vi "Waveform Circular Buffer.vi"(8 "error in":errorcluster, 9 "reset":bool, 10 "buffer duration (s)":dbl=10.0, 11 "waveform in":waveform(dbl)) -> (0 "error out":errorcluster, 3 "waveform out":waveform(dbl))   [LabVIEW 2019, in "DSP.lvclass"]
doc: "Circular buffer for the waveform datatype, designed for use with continuous data acquisition. The output is a single waveform with duration <b>buffer duration (s)</b>, in seconds. Input waveforms are appended to the end of the output waveform, and elements older than the buffer duration are discarded.\n\nAll input waveforms must have matching <i>dt</i> values. To eliminate drift in sample times, only the most recent trigger timestamp is considered; the trigger timestamp of the output waveform is computed from the most recently input trigger timestamp, the duration of the buffer, and <i>dt</i>. This may introduce jitter in sample times if the difference between the final timestamp of the previous input and the trigger timestamp of the next input are not exactly equal to <i>dt</i>. In this case, the timestamps of the most recent portion of the buffer will be correct, but earlier timestamps will be scaled. In buffered continuous acquisition, waveforms are consecutive and no jitter is introduced by this method.\n\nThe duration of the buffer may be larger than the requested duration if the duration is not an integer multiple of <i>dt</i>.\n\nOn first call, the input waveform fills end of the buffer; earlier values are set to zero, and the trigger timestamp is backdated. For performance reasons, <b>buffer duration (s)</b> is read only on first call."
uses:
  DSP.lvclass
  <vilib>/Waveform/WDTOps.llb/WDT Number of Waveform Samples DBL.vi
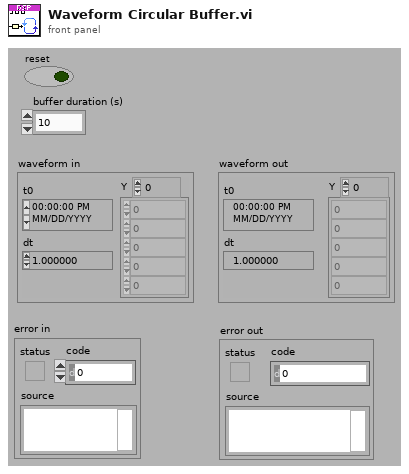
[diagram p1: front panel]
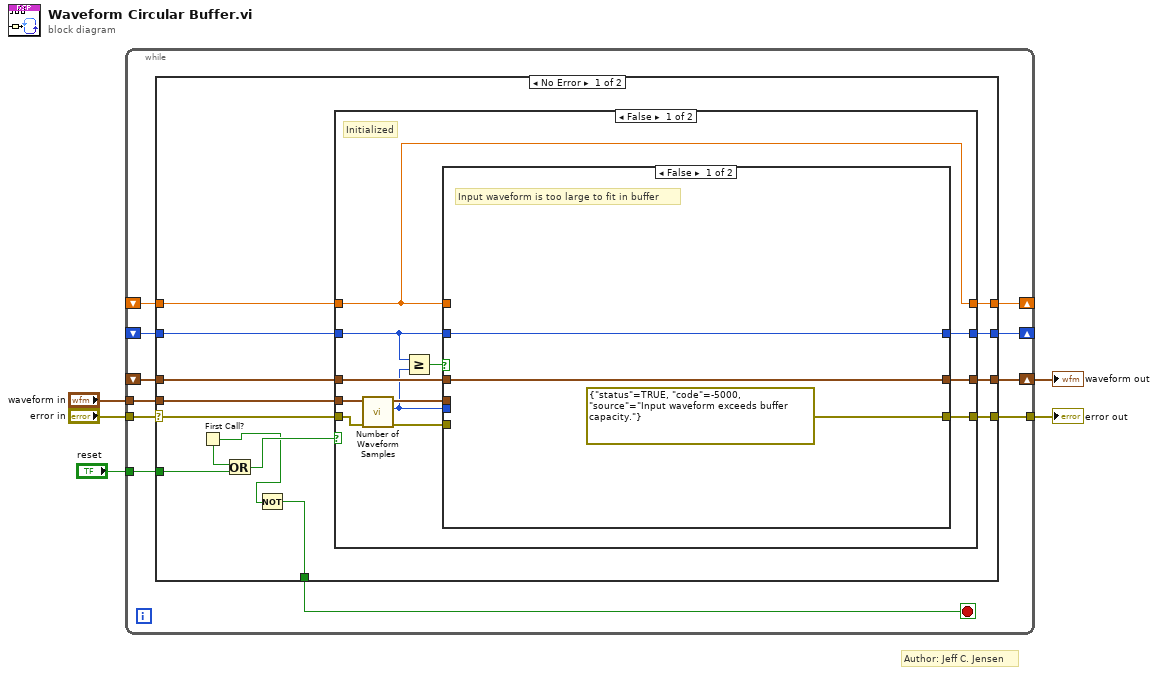
[diagram p0: block diagram]
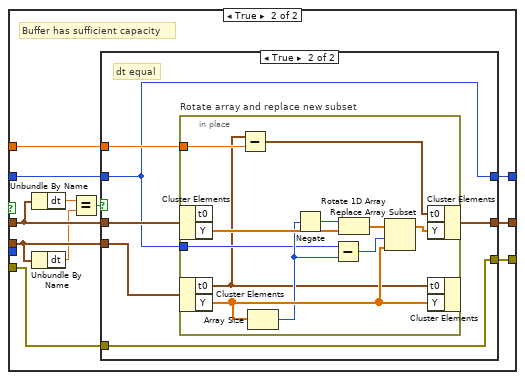
[diagram p2: hidden frame]
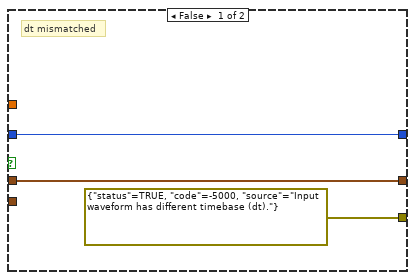
[diagram p3: hidden frame]
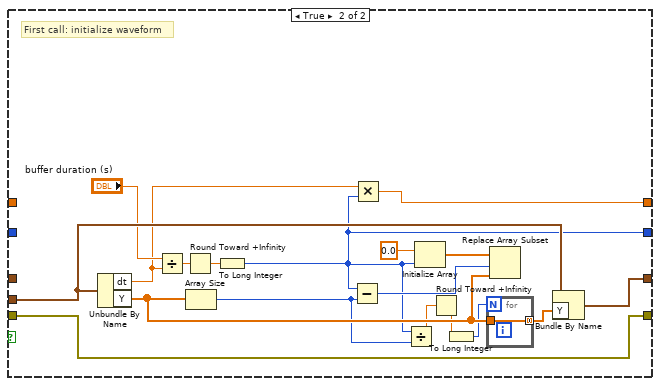
[diagram p4: hidden frame]
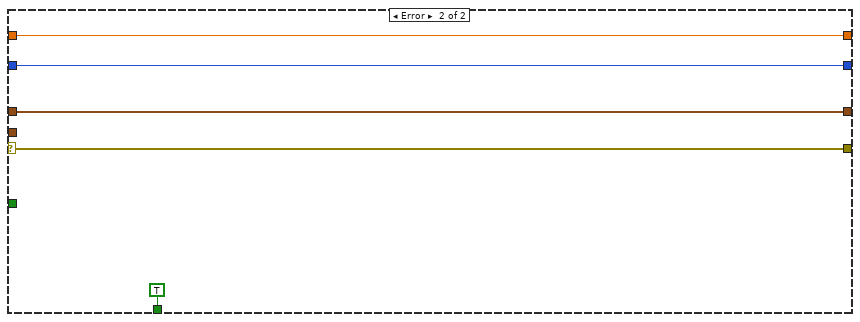
[diagram p5: hidden frame]
diagram:
  # "Author: Jeff C. Jensen"
  n1 = while {
    tunnel: "waveform in" -> [w16]
    tunnel: "error in" -> [w8]
    tunnel: [w14] -> w3
    shift-right: [w15] -> w4
    shift-left: _ -> [w13]
    shift-right: [w12] -> _
    shift-left: _ -> [w11]
    shift-right: [w10] -> _
    shift-left: _ -> [w9]
    tunnel: "reset" -> [w6]
    stop <- w7 stop-if-true
    n2 = case shown="No Error" w8 {
      selector: w8 -> [w21 w95]
      tunnel: w16 -> [w29 _]
      tunnel: [w28 w98] -> w15
      tunnel: [w20 TRUE ("First Call?: T/F")] -> w7
      tunnel: [w27 w95] -> w14
      tunnel: w13 -> [w26 w98]
      tunnel: [w25 w97] -> w12
      tunnel: w11 -> [w24 w97]
      tunnel: [w23 w96] -> w10
      tunnel: w9 -> [w22 w96]
      tunnel: w6 -> [w19 _]
      frame No Error {
        n3 = First Call?() -> (First Call?: T/F=w17:bool)
        n4 = Or(x=w17, y=w19) -> (x .or. y?=w18:bool)
        n5 = Not(x=w17) -> (.not. x?=w20:bool)
        n6 = case shown="False" w18 {
          tunnel: w29 -> [w38 w92]
          tunnel: [w41 w91] -> w28
          tunnel: w21 -> [w37 w90]
          tunnel: [w40 w90] -> w27
          tunnel: w26 -> [w39 _]
          tunnel: [w34 w79] -> w25
          tunnel: w24 -> [w30 _]
          tunnel: [w33 w83] -> w23
          tunnel: w22 -> [w33 _]
          frame False {
            # "Initialized"
            n7 = call-poly <vilib>:"Number of Waveform Samples.vi"("error in (no error)"=w37, "waveform in"=w38) -> ("error out"=w36:errorcluster, "number of samples"=w31:i32, "waveform out"=w35:waveform(dbl))  [unwired: 7 in]
            n8 = Greater Or Equal?(x=w30, y=w31) -> (x >= y?=w32:bool)
            n9 = case shown="False" w32 {
              tunnel: [w44 w55] -> w41
              tunnel: [errorcluster {"status"=TRUE, "code"=-5000, "source"="Input waveform exceeds buffer capacity."} ("error out") w47] -> w40
              tunnel: w39 -> [w44 w51]
              tunnel: w36 -> [_ w46]
              tunnel: w35 -> [_ w52]
              tunnel: w31 -> [_ _]
              tunnel: w30 -> [w43 w54]
              tunnel: [w43 w48] -> w34
              tunnel: w33 -> [_ w53]
              frame False {
                # "Input waveform is too large to fit in buffer"
              }
              frame True {
                # "Buffer has sufficient capacity"
                n10 = Unbundle By Name(w51) -> ("dt"=w50:dbl)
                n11 = Unbundle By Name(w52) -> ("dt"=w49:dbl)
                n12 = Equal?(x=w50, y=w49) -> (x = y?=w45:bool)
                n13 = case shown="True" w45 {
                  tunnel: [w57 w64] -> w55
                  tunnel: w51 -> [w57 w63]
                  tunnel: w52 -> [_ w62]
                  tunnel: w54 -> [w58 w60]
                  tunnel: w53 -> [_ w61]
                  tunnel: [w58 w60] -> w48
                  tunnel: [errorcluster {"status"=TRUE, "code"=-5000, "source"="Input waveform has different timebase (dt)."} ("error out") w59] -> w47
                  tunnel: w46 -> [_ w59]
                  frame False {
                    # "dt mismatched"
                  }
                  frame True {
                    # "dt equal"
                    n14 = in-place "Rotate array and replace new subset" {
                      in-place-border: w60 -> [w68]
                      in-place-border: w61 -> [w66]
                      n15 = in-place-cluster #1(w63) -> ("Y"=w72:dbl[])  [unwired: 1 out]
                      n16 = in-place-cluster #2(w62) -> ("t0"=w65:timestamp, "Y"=w70:dbl[])
                      n17 = Subtract(x=w65, y=w66) -> (x-y=w67:timestamp)
                      n18 = Array Size(array=w70) -> (size(s)=w69:i32)
                      n19 = Negate(x=w69) -> (-x=w73:i32)
                      n20 = Subtract(x=w68, y=w69) -> (x-y=w71:i32)
                      n21 = Rotate 1D Array(1:w72, 2:w73) -> (0:w75:dbl[])
                      n22 = Replace Array Subset(array=w75, new element=w70, index=w71) -> (w74:dbl[])
                      n23 = in-place-cluster #1("t0"=w67, "Y"=w74) -> (w64:waveform(dbl))
                      n24 = in-place-cluster #2("t0"=w65, "Y"=w70) -> ()  [unwired: 1 out]
                    }
                  }
                }
              }
            }
          }
          frame True {
            # "First call: initialize waveform"
            n25 = Unbundle By Name(w92) -> ("dt"=w84:dbl, "Y"=w81:dbl[])
            n26 = Divide(x="buffer duration (s)", y=w84) -> (x/y=w86:dbl)
            n27 = Round Toward +Infinity(x=w86) -> (ceil(x): smallest int >= x=w85:dbl)
            n28 = Array Size(array=w81) -> (size(s)=w80:i32)
            n29 = To Long Integer(number=w85) -> (32bit integer=w79:i32)
            n30 = Subtract(x=w79, y=w80) -> (x-y=w89:i32)
            n31 = Multiply(x=w84, y=w79) -> (x*y=w83:dbl)
            n32 = Divide(x=w79, y=w80) -> (x/y=w78:dbl)
            n33 = Initialize Array(0.0, w79) -> (w88:dbl[])
            n34 = Round Toward +Infinity(x=w78) -> (ceil(x): smallest int >= x=w77:dbl)
            n35 = To Long Integer(number=w77) -> (32bit integer=w76:i32)
            n36 = for {
              N: w76 -> [_]
              tunnel: [w94] -> w82 mode=concatenating
              tunnel: w81 -> [w94]
            }
            n37 = Replace Array Subset(array=w88, new element=w81, index=w89) -> ()  [unwired: 1 out]
            n38 = Bundle By Name(cluster=w92, "Y"=w82) -> (w91:waveform(dbl))
          }
        }
      }
      frame Error {
      }
    }
  }
  "waveform out" <- w4
  "error out" <- w3
